vi "get_use.vi"(3 "error in (no error)":errorcluster, 4 "Remote Server Address":string="palantir", 5 "Target Name":string) -> (0 "error out":errorcluster, 1 "user":string, 2 "in use?":bool)   [LabVIEW 2011]
uses:
  TCPdata.ctl
  TargetData.ctl
panel:
  in  "Cluster":T1
  in  "Listen Port":u16=5311
  in  "Remote Server Port":u16=5310
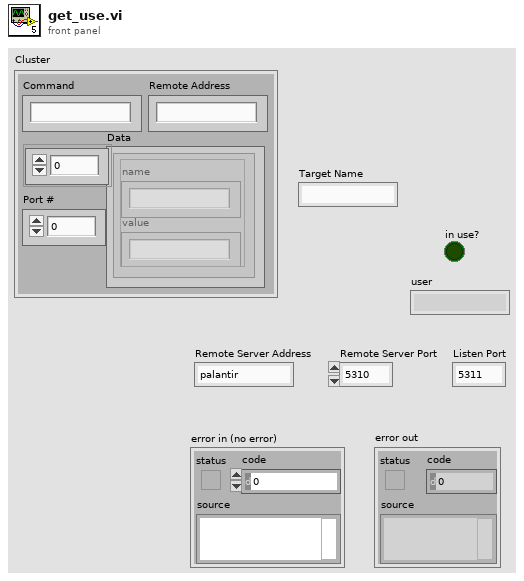
[diagram p1: front panel]
types:
  T1 = typedef "TCPdata.ctl" = cluster{"Data":T2, "Command":string, "Remote Address":string, "Port #":u16}
  T2 = typedef "TargetData.ctl" = cluster{"name":string, "value":string}[]
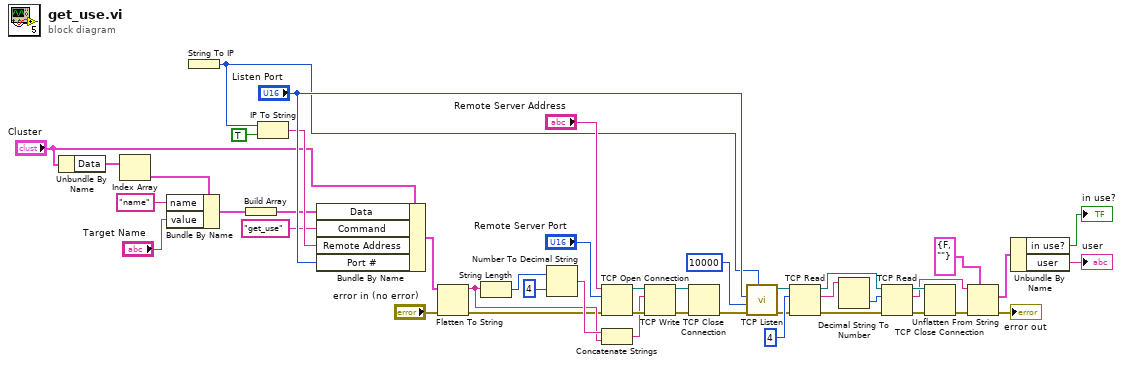
[diagram p0: block diagram]
diagram:
  n1 = Unbundle By Name("Cluster") -> ("Data"=w29:T2)
  n2 = Index Array(array=w29) -> (element=w28:cluster{"name":string, "value":string})  [unwired: 1 in]
  n3 = Bundle By Name(cluster=w28, "name"="name", "value"="Target Name") -> (w27:cluster{"name":string, "value":string})
  n4 = String To IP() -> (0:w21:u32)  [unwired: 1 in]
  n5 = Build Array(w27) -> (w26:cluster{"name":string, "value":string}[])
  n6 = IP To String(1:TRUE ("dot notation? (F)"), 2:w21) -> (0:w32:string)
  n7 = Bundle By Name(cluster="Cluster", "Data"=w26, "Command"="get_use", "Remote Address"=w32, "Port #"="Listen Port") -> (w16:T1)
  n8 = Flatten To String(anything=w16, error in (no error)="error in (no error)") -> (data string=w15:string, error out=w13:errorcluster)  [unwired: 2 in, 1 out]
  n9 = String Length(string=w15) -> (length=w19:i32)
  n10 = Number To Decimal String(number=w19, width (-)=i16 4) -> (decimal integer string=w18:string)
  n11 = TCP Open Connection(address="Remote Server Address", remote port or service name="Remote Server Port", error in (no error)=w13) -> (connection ID=w44:refnum<k5>, error out=w43:errorcluster)  [unwired: 2 out]
  n12 = Concatenate Strings(w18, w15) -> (w20:string)
  n13 = TCP Write(connection ID=w44, data in=w20, error in (no error)=w43) -> (connection ID out=w41:refnum<k5>, error out=w42:errorcluster)  [unwired: 2 out]
  n14 = TCP Close Connection(connection ID=w41, error in (no error)=w42) -> (error out=w35:errorcluster)  [unwired: 2 out]
  n15 = call <vilib>:"TCP Listen.vi"("net address"=w21, "error in (no error)"=w35, "timeout ms (wait forever: -1)"=10000, "port"="Listen Port") -> ("error out"=w10:errorcluster, "connection ID"=w8:refnum<k5>)  [unwired: 3 in, 3 out]
  n16 = TCP Read(connection ID=w8, bytes to read=4, error in (no error)=w10) -> (connection ID out=w7:refnum<k5>, data out=w11:string, error out=w9:errorcluster)  [unwired: 1 in, 1 out]
  n17 = Decimal String To Number(string=w11) -> (number=w6:i32)  [unwired: 2 in, 1 out]
  n18 = TCP Read(connection ID=w7, bytes to read=w6, error in (no error)=w9) -> (connection ID out=w38:refnum<k5>, data out=w4:string, error out=w36:errorcluster)  [unwired: 1 in, 1 out]
  n19 = TCP Close Connection(connection ID=w38, error in (no error)=w36) -> (error out=w5:errorcluster)  [unwired: 2 out]
  n20 = Unflatten From String(type=cluster{"in use?":bool, "user":string} {"in use?"=FALSE, "user"=""} ("output cluster"), binary string=w4, error in (no error)=w5) -> (value=w1:cluster{"in use?":bool, "user":string}, error out=→"error out":errorcluster)  [unwired: 2 in, 1 out]
  n21 = Unbundle By Name(w1) -> ("in use?"=→"in use?":bool, "user"=→"user":string)
